vi "Get UI Ref.vi"(8 "error in (no error)":errorcluster, 11 "9235 in":refnum<class "9235.lvclass">) -> (0 "error out":errorcluster, 1 "Show SubPanel?":bool, 2 "VI Refnum":refnum<vi>, 3 "9235 out":refnum<class "9235.lvclass">)   [LabVIEW 2020, in "Modules.lvlib" / "9235.lvclass"]
uses:
  9235.lvclass
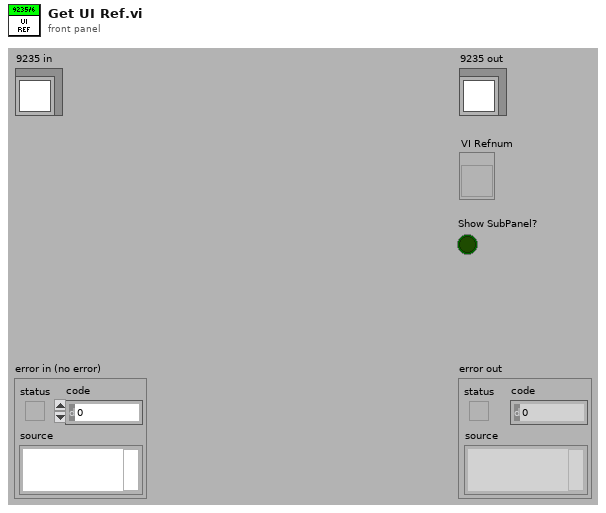
[diagram p1: front panel]
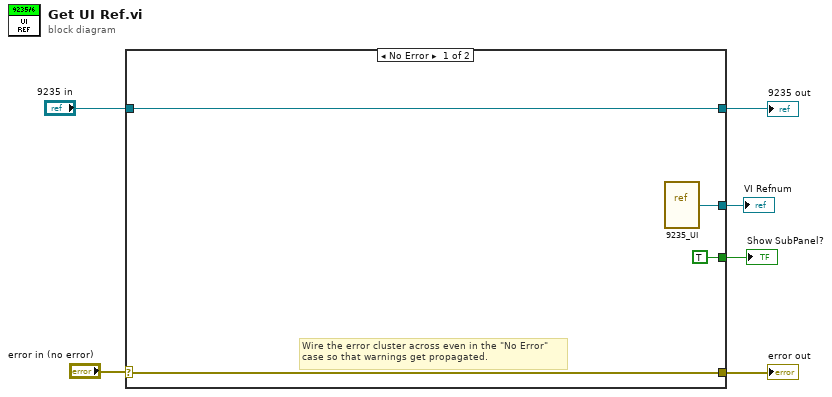
[diagram p0: block diagram]
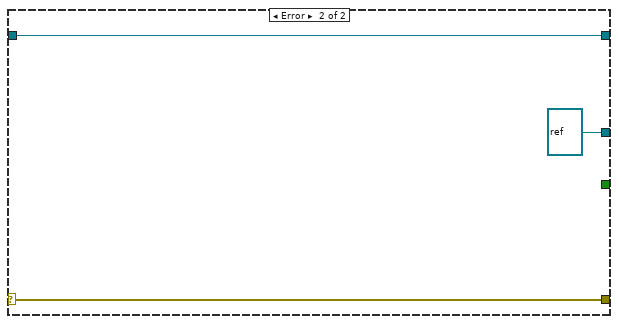
[diagram p2: hidden frame]
diagram:
  n1 = case shown="No Error" "error in (no error)" {
    selector: "error in (no error)" -> [w9 w13]
    tunnel: [w9 w13] -> w3
    tunnel: [w10 w12] -> w5
    tunnel: "9235 in" -> [w10 w12]
    tunnel: [w8 refnum<vi> refnum] -> w2
    tunnel: [TRUE _] -> w1
    frame No Error {
      # "Wire the error cluster across even in the \"No Error\"\ncase so that warnings get propagated."
      n2 = vi-ref "9235_UI.vi"() -> (w8:refnum<vi>)
    }
    frame Error {
    }
  }
  "error out" <- w3
  "9235 out" <- w5
  "VI Refnum" <- w2
  "Show SubPanel?" <- w1
